vi "ma_SML Adjacent Channel Power.vi"(6 "impedance(ohm)":dbl=50.0 format="%.2f", 7 "units [rms]":T2(ring)=enum."V^2", 8 "error in (no error)":errorcluster, 9 "channel":T3 {"spacing" format="%.2f"; "bandwidth" format="%.2f"; "center frequency" format="%.2f"}, 10 "spectral info":T1 {"window" items=["Rectangle"=0, "Hanning"=1, "Hamming"=2, "Blackman-Harris"=3, "Exact Blackman"=4, "Blackman"=5, "Flat Top"=6, "4 Term B-Harris "=7, "7 Term B-Harris"=8, "Low Sidelobe"=9, "Blackman Nuttall"=11, "Triangle"=30, "Bartlett-Hanning"=31, "Bohman"=32, "Parzen"=33, "Welch"=34, "Kaiser"=60, "Dolph-Chebyshev"=61, "Gaussian"=62]}, 11 "power spectrum":T4 {"spectrum" format="%.2f"; "df" format="%.2f"; "f0" format="%.2f"}) -> (0 "error out":errorcluster, 1 "power in lower channel":dbl format="%.2f", 2 "power in upper channel":dbl format="%.2f", 3 "power in channel":dbl format="%.2f", 4 "units string":string)   [LabVIEW 2020, in "NI_MAPro.lvlib"]
uses:
  NI_MAPro.lvlib
  ma_sml_Spectrum Cluster (real).ctl
  ma_sml_Spectral Info.ctl
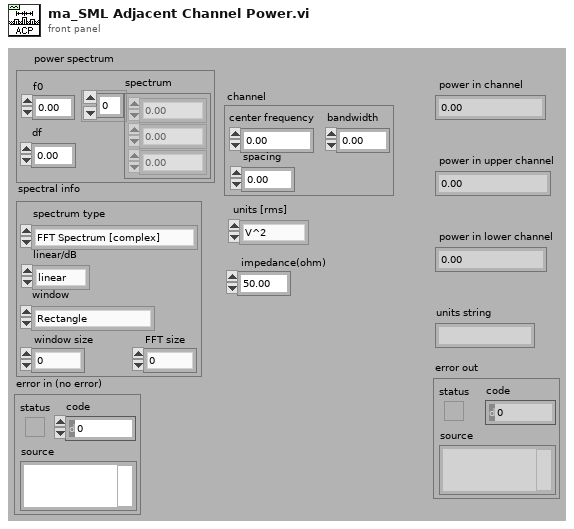
[diagram p1: front panel]
types:
  T1 = typedef "NI_MAPro.lvlib/ma_sml_Spectral Info.ctl" = cluster{"spectrum type":enum16{"FFT Spectrum [complex]", "Amplitude [Magnitude]", "Power [Magnitude^2]", "Cross Spectrum [complex]", "Frequency Response [Complex]"}, "linear/dB":enum16{"linear", "dB"}, "window":u16, "window size":i32, "FFT size":i32}
  T2 = enum16{"V", "V^2", "W", "dBm", "dBW", "dBV", "dBmV", "dBuV"}
  T3 = cluster{"center frequency":dbl, "bandwidth":dbl, "spacing":dbl}
  T4 = typedef "NI_MAPro.lvlib/ma_sml_Spectrum Cluster (real).ctl" = cluster{"f0":dbl, "df":dbl, "spectrum":dbl[]}
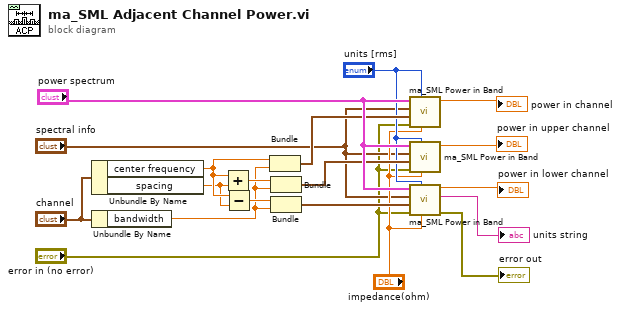
[diagram p0: block diagram]
diagram:
  n1 = Unbundle By Name("channel") -> ("center frequency"=w16:dbl, "spacing"=w15:dbl)
  n2 = Unbundle By Name("channel") -> ("bandwidth"=w12:dbl)
  n3 = Add(x=w16, y=w15) -> (x+y=w14:dbl)
  n4 = Subtract(x=w16, y=w15) -> (x-y=w13:dbl)
  n5 = Bundle("center frequency"=w16, "bandwidth"=w12) -> (w17:cluster{"center frequency":dbl, "bandwidth":dbl})  [unwired: 1 out]
  n6 = Bundle(w14, "bandwidth"=w12) -> (w11:cluster{dbl, "bandwidth":dbl})  [unwired: 1 out]
  n7 = Bundle(w13, "bandwidth"=w12) -> (w10:cluster{dbl, "bandwidth":dbl})  [unwired: 1 out]
  n8 = call "ma_SML Power in Band.vi"("impedance(ohm)"="impedance(ohm)", "units [rms]"="units [rms]", "error in (no error)"="error in (no error)", "band"=w17, "spectral info"="spectral info", "power spectrum"="power spectrum") -> ("power in band"=→"power in channel":dbl)  [unwired: 5 out]
  n9 = call "ma_SML Power in Band.vi"("impedance(ohm)"="impedance(ohm)", "units [rms]"="units [rms]", "error in (no error)"="error in (no error)", "band"=w11, "spectral info"="spectral info", "power spectrum"="power spectrum") -> ("power in band"=→"power in upper channel":dbl)  [unwired: 5 out]
  n10 = call "ma_SML Power in Band.vi"("impedance(ohm)"="impedance(ohm)", "units [rms]"="units [rms]", "error in (no error)"="error in (no error)", "band"=w10, "spectral info"="spectral info", "power spectrum"="power spectrum") -> ("error out"=→"error out":errorcluster, "units string"=→"units string":string, "power in band"=→"power in lower channel":dbl)  [unwired: 3 out]
